vi "GEOM_CorrXcoord_dataonly.vi"(10 "levels":cluster{"amplifiers":i32, "coord":i32}[](array[cluster]), 11 "Array":T1[](array[typedef]) {"fliped" items=["none", "horizontal", "vertical"]; "type" items=["LL", "LR", "UL", "UR"]}) -> (1 "xcoord":u32, 3 "Array 2":T1[](array[typedef]) {"fliped" items=["none", "horizontal", "vertical"]; "type" items=["LL", "LR", "UL", "UR"]})   [LabVIEW 2016]
uses:
  GEOM_Amplifier.ctl
  GEOM_AmpType.ctl
  GEOM_ROI.ctl
  GEOM_Coords.ctl
panel:
  out "maxx":u32
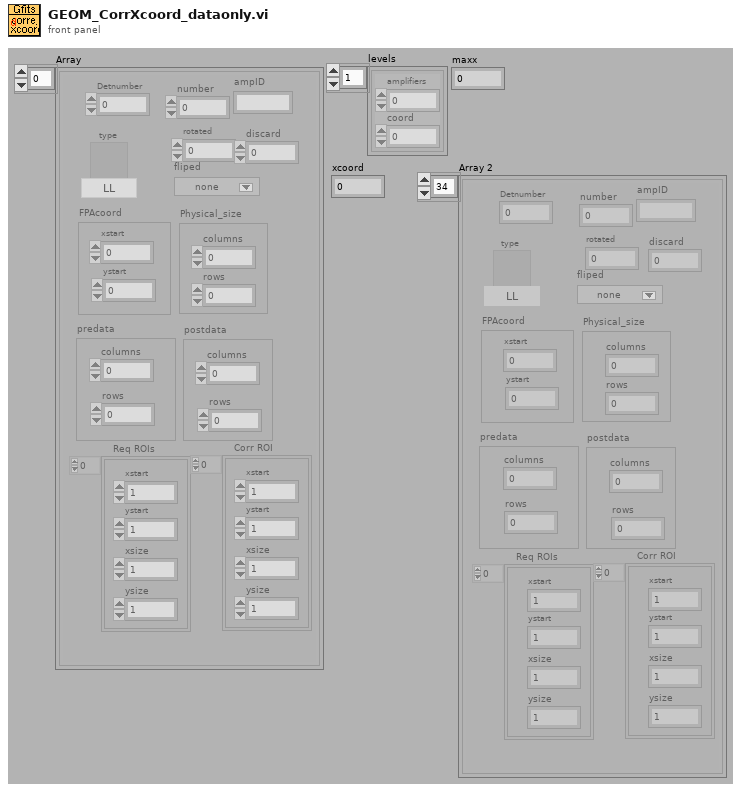
[diagram p1: front panel]
types:
  T1 = typedef "GEOM_Amplifier.ctl" = cluster{"number":i32, "type":T2, "rotated":i16, "fliped":u16, "FPAcoord":cluster{"xstart":i32, "ystart":i32}, "Physical_size":cluster{"columns":i32, "rows":i32}, "predata":cluster{"columns":i32, "rows":i32}, "postdata":cluster{"columns":i32, "rows":i32}, "Req ROIs":T3, "Corr ROI":T3, "Detnumber":i32, "ampID":string, "discard":i32}
  T2 = typedef "GEOM_AmpType.ctl" = u16
  T3 = typedef "GEOM_ROI.ctl" = T4[]
  T4 = typedef "GEOM_Coords.ctl" = cluster{"xstart":u32, "ystart":u32, "xsize":u32, "ysize":u32}
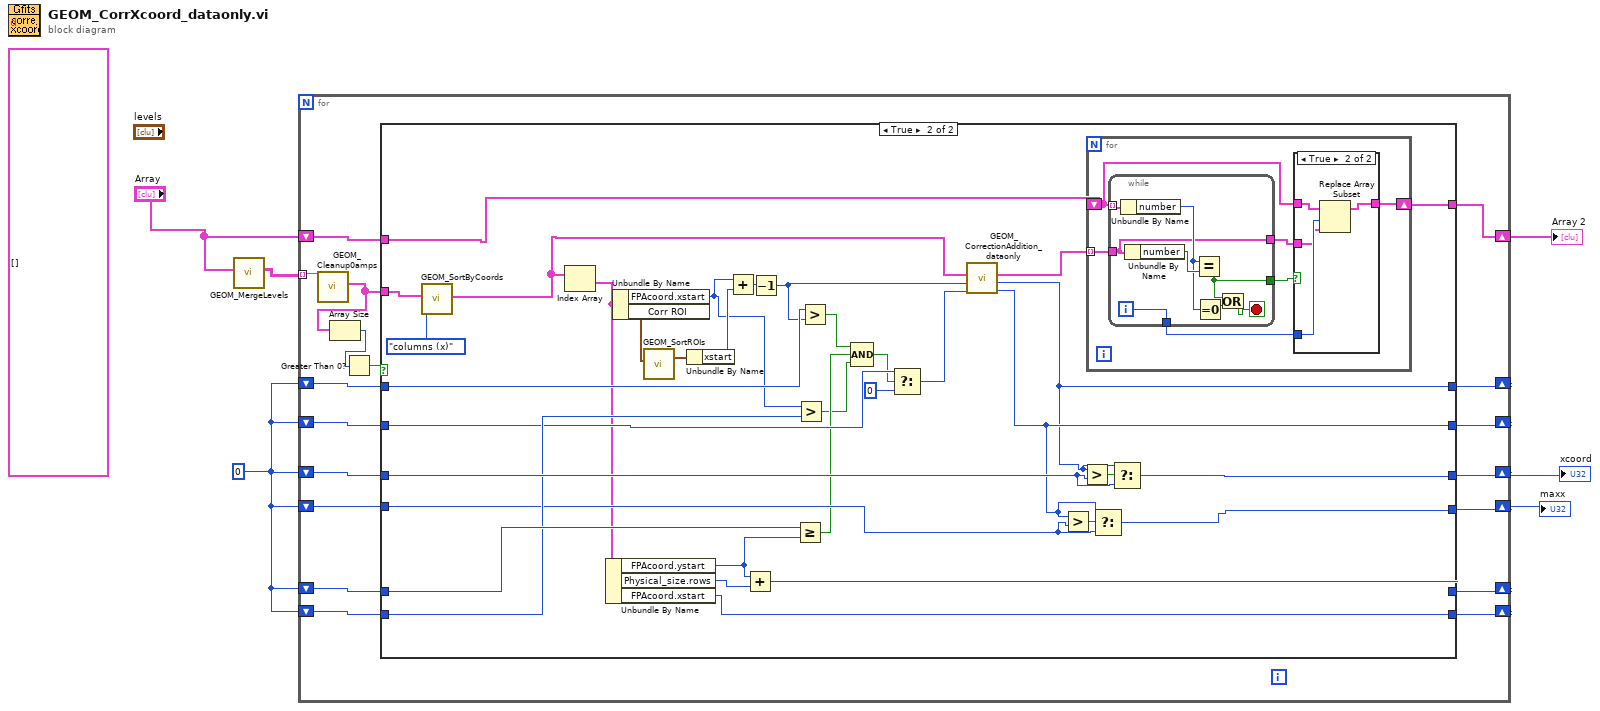
[diagram p0: block diagram]
diagram:
  (unwired) T1[] []
  w4 = u32 0
  n1 = call "GEOM_MergeLevels.vi"("Array"="Array") -> ("amplifiers 2"=w1:T1[][])  [unwired: 10 out]
  n2 = for {
    shift-right: [w11] -> w3
    shift-left: "Array" -> [w12]
    shift-right: [w24] -> w6
    shift-left: w4 -> [w23]
    shift-right: [w22] -> w5
    shift-left: w4 -> [w14]
    shift-right: [w20] -> _
    shift-left: w4 -> [w21]
    shift-right: [w19] -> _
    shift-left: w4 -> [w18]
    shift-right: [w17] -> _
    shift-left: w4 -> [w16]
    shift-right: [w15] -> _
    shift-left: w4 -> [w13]
    tunnel: w1 -> [w10] mode=indexing
    n3 = call "GEOM_Cleanup0amps.vi"("sorted amplifiers"=w10) -> ("amps out"=w9:T1[])  [unwired: 10 out]
    n4 = Array Size(array=w9) -> (size(s)=w8:i32)
    n5 = Greater Than 0?(x=w8) -> (x > 0?=w7:bool)
    n6 = case shown="True" w7 {
      tunnel: [w29 w66] -> w24
      tunnel: w23 -> [w29 w65]
      tunnel: [w28 w64] -> w22
      tunnel: w21 -> [w27 w63]
      tunnel: [w27 w62] -> w20
      tunnel: [w31 w34] -> w19
      tunnel: w18 -> [w31 w61]
      tunnel: [w26 w60] -> w17
      tunnel: w16 -> [w26 w59]
      tunnel: [w30 w35] -> w15
      tunnel: w14 -> [w28 w58]
      tunnel: w13 -> [w30 w57]
      tunnel: w12 -> [w25 w55]
      tunnel: [w25 w54] -> w11
      tunnel: w9 -> [_ w38]
      frame False {
      }
      frame True {
        n7 = call "GEOM_SortByCoords.vi"("amplifiers"=w38, "how"=enum16{"rows (y)", "columns (x)"}."columns (x)") -> ("sorted amplifiers"=w37:T1[])  [unwired: 9 out]
        n8 = Index Array(array=w37) -> (element=w53:T1)  [unwired: 1 in]
        n9 = Unbundle By Name(w53) -> ("FPAcoord.ystart"=w44:i32, "Physical_size.rows"=w46:i32, "FPAcoord.xstart"=w60:i32)
        n10 = Unbundle By Name(w53) -> ("FPAcoord.xstart"=w42:i32, "Corr ROI"=w51:T3)
        n11 = call "GEOM_SortROIs.vi"("ROIs"=w51) -> ("Extreme Coords"=w50:T4)  [unwired: 10 out]
        n12 = Unbundle By Name(w50) -> ("xstart"=w47:u32)
        n13 = Add(x=w42, y=w47) -> (x+y=w49:u32)
        n14 = Add(x=w44, y=w46) -> (x+y=w62:i32)
        n15 = Decrement(x=w49) -> (x-1=w32:u32)
        n16 = Greater Or Equal?(x=w63, y=w44) -> (x >= y?=w45:bool)
        n17 = Greater?(x=w42, y=w59) -> (0:w43:bool)
        n18 = Greater?(x=w61, y=w32) -> (0:w39:bool)
        n19 = Compound Arithmetic op=AND(w39, w45, w43) -> (w41:bool)
        n20 = Select(t=w57, s=w41, f=u32 0) -> (s? t:f=w36:u32)
        n21 = call "GEOM_CorrectionAddition_dataonly.vi"("ini shift"=w36, "iniX"=w32, "sorted amplifiers"=w37) -> ("out shift"=w35:u32, "out x"=w34:u32, "amplifiers out"=w33:T1[])  [unwired: 6 out]
        n22 = Greater?(x=w35, y=w58) -> (0:w48:bool)
        n23 = Greater?(x=w34, y=w65) -> (0:w52:bool)
        n24 = for {
          tunnel: w33 -> [w72] mode=indexing
          shift-right: [w68] -> w54
          shift-left: w55 -> [w69]
          n25 = while {
            tunnel: w69 -> [w85] mode=indexing
            tunnel: w72 -> [w80]
            tunnel: [w81] -> w71
            tunnel: [w80] -> w70
            tunnel: [w79] -> w67
            i -> [w79]
            stop <- w78 stop-if-true
            n26 = Unbundle By Name(w85) -> ("number"=w83:i32)
            n27 = Unbundle By Name(w80) -> ("number"=w84:i32)
            n28 = Equal?(x=w83, y=w84) -> (x = y?=w81:bool)
            n29 = Equal To 0?(x=w83) -> (x = 0?=w82:bool)
            n30 = Or(x=w81, y=w82) -> (x .or. y?=w78:bool)
          }
          n31 = case shown="True" w71 {
            tunnel: w70 -> [_ w74]
            tunnel: w69 -> [w73 w77]
            tunnel: [w73 w76] -> w68
            tunnel: w67 -> [_ w75]
            frame False {
            }
            frame True {
              n32 = Replace Array Subset(array=w77, new element=w74, index=w75) -> (w76:T1[])
            }
          }
        }
        n33 = Select(t=w35, s=w48, f=w58) -> (s? t:f=w64:u32)
        n34 = Select(t=w34, s=w52, f=w65) -> (s? t:f=w66:u32)
      }
    }
  }
  "Array 2" <- w3
  "xcoord" <- w6
  "maxx" <- w5
